vi "Editor.vi"(9 "Editor Events":T11, 11 "VIDoc Settings - Confluence In":refnum<class "VIDoc Settings - Confluence.lvclass">) -> (3 "VIDoc Settings - Confluence Out":refnum<class "VIDoc Settings - Confluence.lvclass">)   [LabVIEW 2023, in "VIDoc Printer - Confluence.lvlib" / "VIDoc Settings - Confluence.lvclass"]
uses:
  VIDoc Settings - Confluence.lvclass
  Interfaces/VIDoc Editor/Editor Events Cluster.ctl
  Confluence Connection Settings.ctl
  Class Info Column.ctl
  VI Info Column.ctl
  Control Info Column.ctl
  VIDoc Settings - Confluence.lvclass/VIDoc Settings - Confluence.ctl
  <userlib>/_PetranWay/LabVIEW Confluence API/Source/Data Center/Confluence Data Center/Confluence Data Center.lvclass
  C:/Program Files/National Instruments/LabVIEW 2023/user.lib/_PetranWay/LabVIEW Confluence API/Source/Confluence/Confluence Connection/Confluence.lvclass
  <userlib>/_PetranWay/LabVIEW Confluence API/Source/Cloud/Confluence Cloud/Confluence Cloud.lvclass
  <userlib>/_PetranWay/LabVIEW Confluence API/Source/Data Center/Confluence Data Center/API/Construct Confluence Data Center From Cache.vi
  <userlib>/_PetranWay/LabVIEW Confluence API/Source/Cloud/Confluence Cloud/API/Construct Confluence Cloud From Cache.vi
  <userlib>/_PetranWay/LabVIEW Confluence API/Source/Confluence/Confluence Connection/Confluence.lvclass
  Interfaces/VIDoc Editor/VIDocEditor.lvclass
panel:
  in  "Sections Tabs":T1(tab)
  out "Connection?":bool
  in  "Test Confluence Connection":bool
  in  "Sortable Tables":bool=TRUE
  in  "Confluence Connection Settings":T2
  in  "Expand Structures":T3={"VI Member"={"By Folder Expand"=TRUE, "By Tree Expand"=TRUE, "By List Expand"=TRUE, "Methods Expand"=TRUE, "Controls Expand"=TRUE}, "Control Member"={"By Folder Expand"=TRUE, "By Tree Expand"=TRUE, "By List Expand"=TRUE, "Controls Expand"=TRUE}, "Interface"={"List Expand"=TRUE, "Controls Expand"=TRUE, "Methods Expand"=TRUE, "Inheritance Expand"=TRUE}, "Library"={"By Folder Expand"=TRUE, "By Tree Expand"=TRUE, "By List Expand"=TRUE, "Controls Expand"=TRUE, "Methods Expand"=TRUE, "Inheritance Expand"=TRUE}, "Class"={"By Folder Expand"=TRUE, "By Tree Expand"=TRUE, "By List Expand"=TRUE, "CPD Expand"=TRUE, "Controls Expand"=TRUE, "Methods Expand"=TRUE, "Set Accessors Expand"=TRUE, "Get Accessors Expand"=TRUE, "Inheritance Expand"=TRUE}}
  in  "Table Column Ordering":T4(tab)
  in  "Class List":T6
  in  "Library List":T6
  in  "Method List":T8
  in  "Interface Methods":T8
  in  "Library Methods":T8
  in  "Class Methods":T8
  in  "LLB Methods":T8
  in  "UI Methods":T8
  in  "Library Control Files":T8
  in  "Control FP":T10
  # "Effects:\nClass - By List\nClass - Inheritance Parent Class\nClass - Inheritance Parent Interfaces\nInterface - By List\nInterface - Inheritance Parent Interfaces"
  # "Effects:\nClass - Inheritance Parent Libraries\nLibrary - By List"
  # "Effects:\nControls - By List\nUI - By List"
  # "Effects:\nInterface - Methods"
  # "Effects:\nLibrary - Methods"
  # "Effects:\nGet Accessors\nSet Accessors\nClass - Methods"
  # "Effects:\nLLB - Methods"
  # "Effects:\nUI - Method Details"
  # "Effects:\nClass - Controls\nInterface - Controls\nLibrary - Controls\nLLB - Controls"
  # "Effects:\nClass - CPD\nControls - Controls\nUI - Controls"
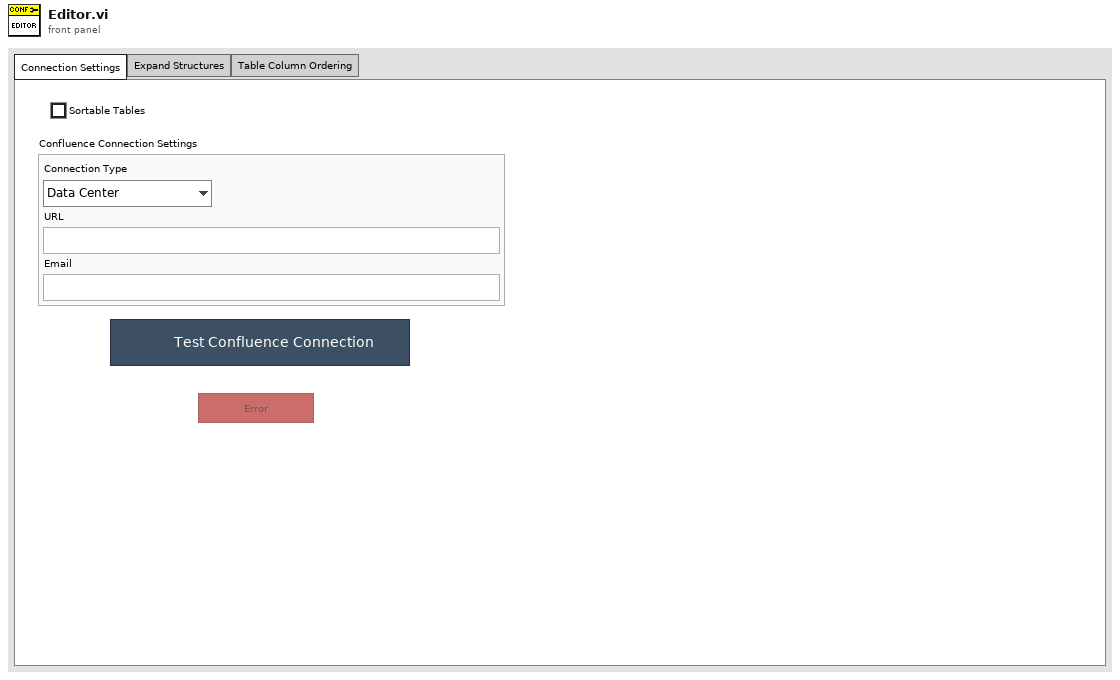
[diagram p1: front panel]
types:
  T1 = enum32{"Connection Settings", "Expand Structures", "Table Column Ordering"}
  T2 = typedef "VIDoc Printer - Confluence.lvlib/VIDoc Settings - Confluence.lvclass/Confluence Connection Settings.ctl" = cluster{"Connection Type":enum16{"Data Center", "Cloud"}, "URL":string, "Email":string}
  T3 = cluster{"VI Member":cluster{"By Folder Expand":bool, "By Tree Expand":bool, "By List Expand":bool, "Methods Expand":bool, "Controls Expand":bool}, "Control Member":cluster{"By Folder Expand":bool, "By Tree Expand":bool, "By List Expand":bool, "Controls Expand":bool}, "Interface":cluster{"List Expand":bool, "Controls Expand":bool, "Methods Expand":bool, "Inheritance Expand":bool}, "Library":cluster{"By Folder Expand":bool, "By Tree Expand":bool, "By List Expand":bool, "Controls Expand":bool, "Methods Expand":bool, "Inheritance Expand":bool}, "Class":cluster{"By Folder Expand":bool, "By Tree Expand":bool, "By List Expand":bool, "CPD Expand":bool, "Controls Expand":bool, "Methods Expand":bool, "Set Accessors Expand":bool, "Get Accessors Expand":bool, "Inheritance Expand":bool}}
  T4 = enum32{"Class List", "Library List", "Methods List", "Interface Methods", "Library Methods", "Class Methods", "LLB Methods", "UI Methods", "Library Control Files", "Font Panel Controls"}
  T5 = typedef "VIDoc Printer - Confluence.lvlib/VIDoc Settings - Confluence.lvclass/Class Info Column.ctl" = enum16{"Image", "Name", "Description", "Version", "Last Change", "Author", "Commit Hash", "Branch", "Qualified Name", "TransferMustOverrides", "ChildRefsRestricted"}
  T6 = cluster{"Minimal":T5[], "Standard":T5[], "Full":T5[]}
  T7 = typedef "VIDoc Printer - Confluence.lvlib/VIDoc Settings - Confluence.lvclass/VI Info Column.ctl" = enum16{"Name", "Conpane", "BD", "FP", "VI Icon", "Description", "Reentrant", "Inline", "Auto Error", "Compiled", "Code Complexity", "Data Size", "Debug", "Priority", "Rev", "Minimum Size", "Title", "FP Behavior", "FP Closeable", "Author", "Commit Hash", "Last Change", "Branch", "Scope", "Type", "Dispatch", "Must Override", "Must Use Parent", "Structure Tree"}
  T8 = cluster{"Minimal":T7[], "Standard":T7[], "Full":T7[]}
  T9 = typedef "VIDoc Printer - Confluence.lvlib/VIDoc Settings - Confluence.lvclass/Control Info Column.ctl" = enum16{"Image", "Name", "Description", "Caption", "Tip Strip", "Data Type", "Key Toggle"}
  T10 = cluster{"Minimal":T9[], "Standard":T9[], "Full":T9[]}
  T11 = typedef "VIDocEditor.lvclass/Editor Events Cluster.ctl" = cluster{"Close":refnum<user-event>, "Revert":refnum<user-event>, "Save":refnum<user-event>, "Changes?":refnum<user-event>}
  T12 = enum8{"Enabled", "Disabled", "Disabled and Grayed Out"}
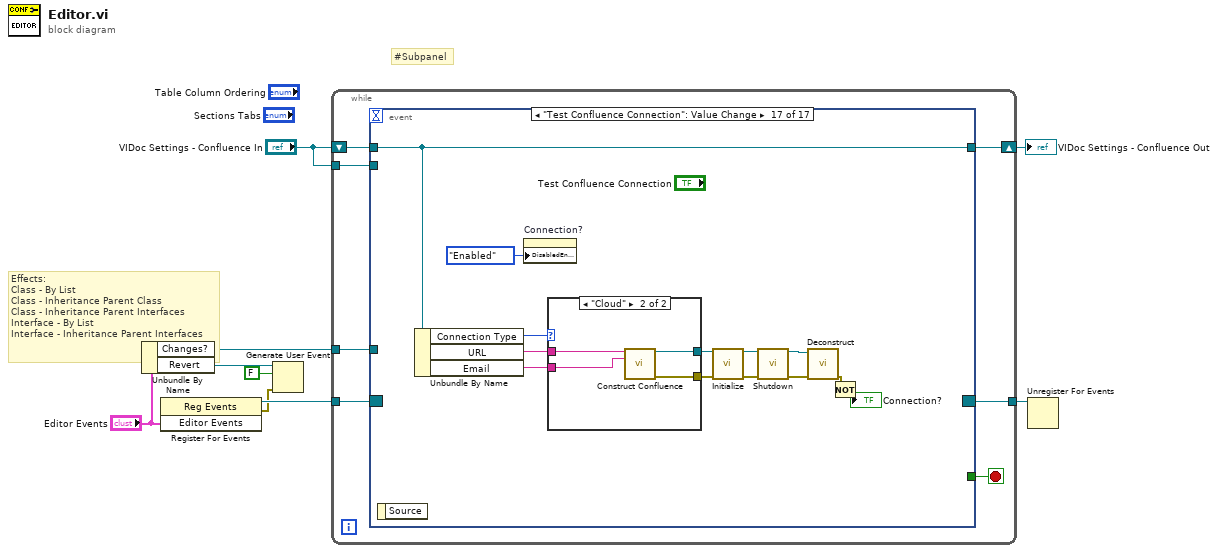
[diagram p0: block diagram]
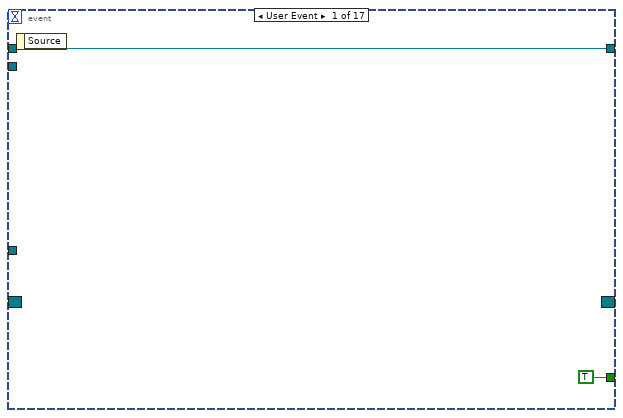
[diagram p2: hidden frame]
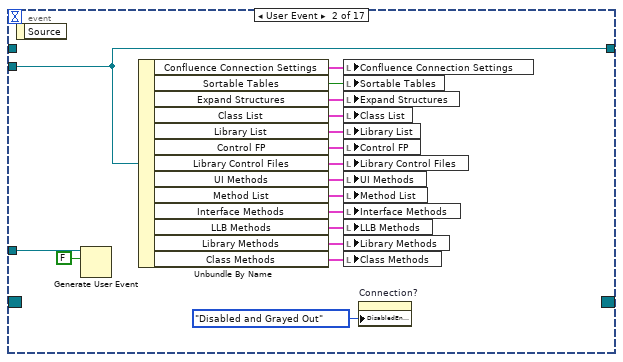
[diagram p3: hidden frame]
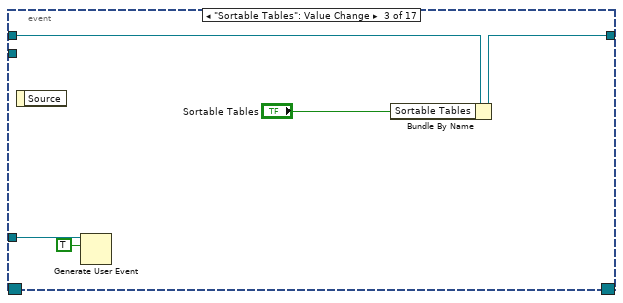
[diagram p4: hidden frame]
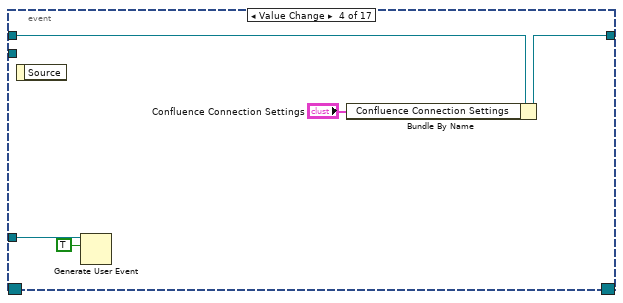
[diagram p5: hidden frame]
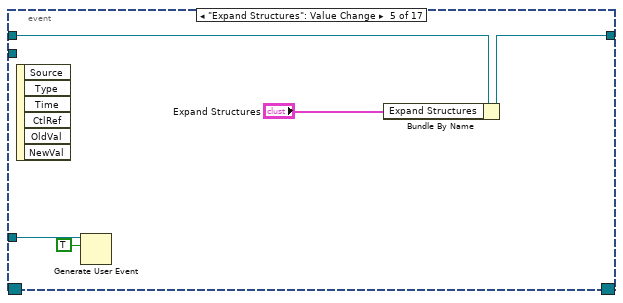
[diagram p6: hidden frame]
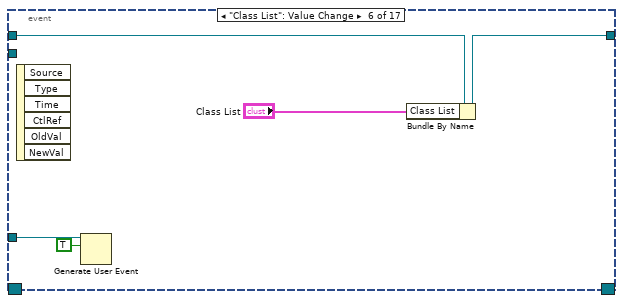
[diagram p7: hidden frame]
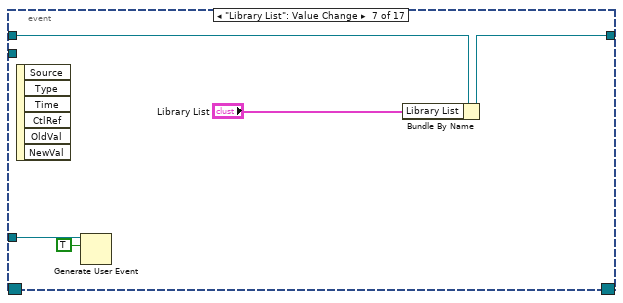
[diagram p8: hidden frame]
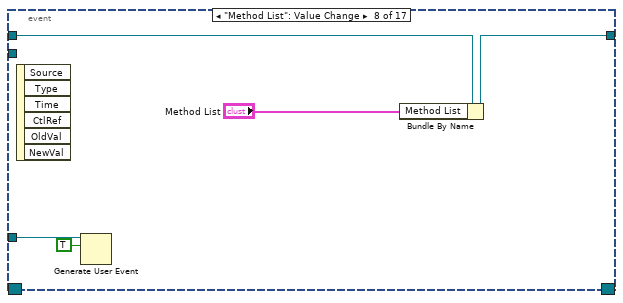
[diagram p9: hidden frame]
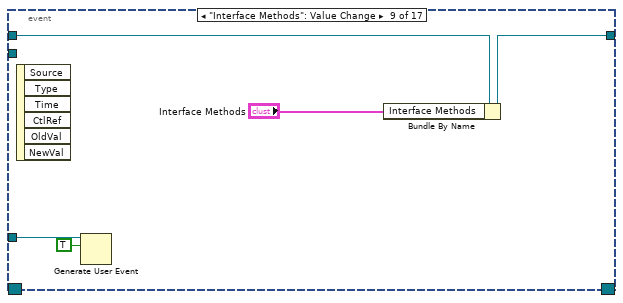
[diagram p10: hidden frame]
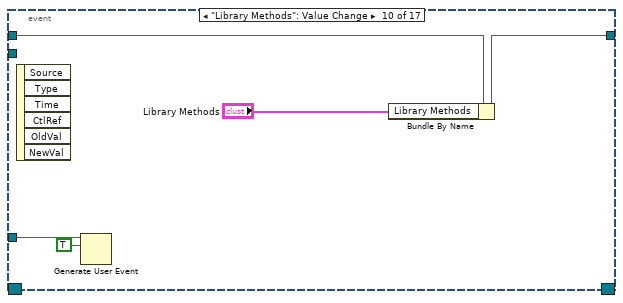
[diagram p11: hidden frame]
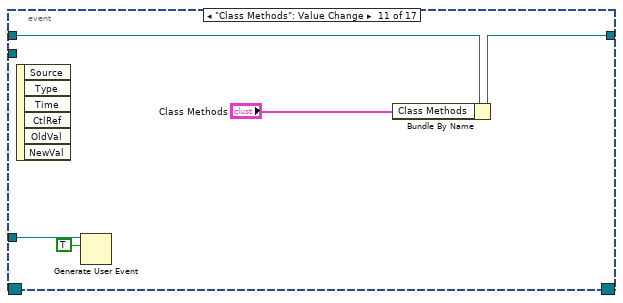
[diagram p12: hidden frame]
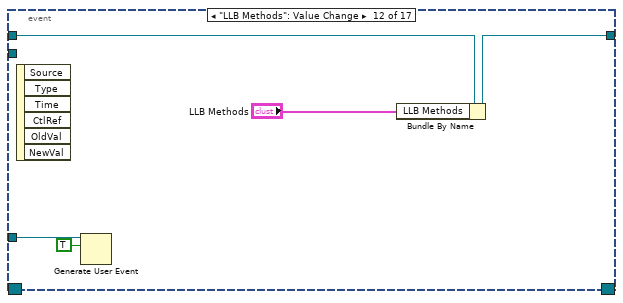
[diagram p13: hidden frame]
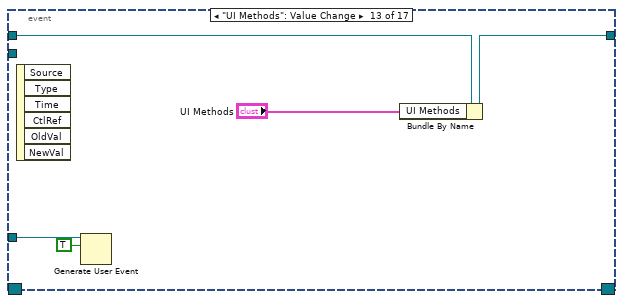
[diagram p14: hidden frame]
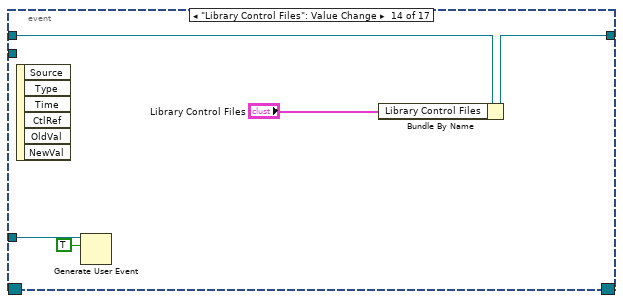
[diagram p15: hidden frame]
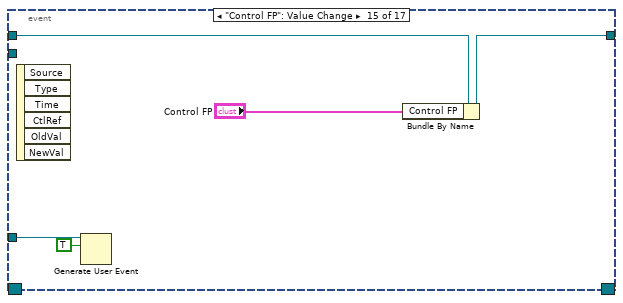
[diagram p16: hidden frame]
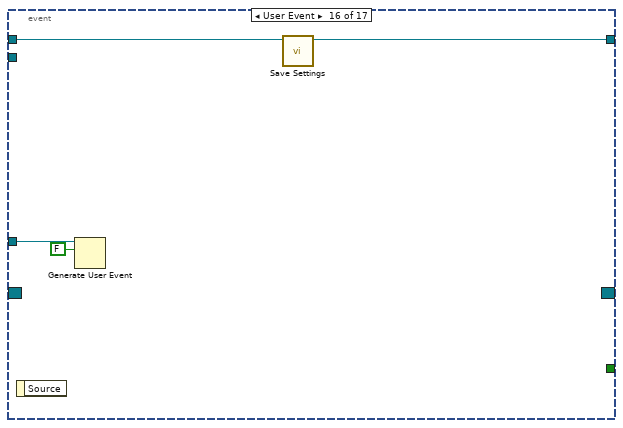
[diagram p17: hidden frame]
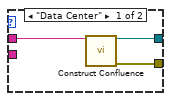
[diagram p18: hidden frame]
diagram:
  # "#Subpanel"
  # "Effects:\nClass - By List\nClass - Inheritance Parent Class\nClass - Inheritance Parent Interfaces\nInterface - By List\nInterface - Inheritance Parent Interfaces"
  n1 = Unbundle By Name("Editor Events") -> ("Changes?"=w1:refnum<user-event>, "Revert"=w4:refnum<user-event>)
  n2 = register-events("Editor Events") -> (reference out=w9:refnum<event-registration>, error out=w2:errorcluster)  [unwired: 2 in]
  n3 = Generate User Event(user event=w4, event data cluster=FALSE ("event data"), error in=w2) -> ()  [unwired: 1 in, 2 out]
  n4 = while {
    shift-right: [w14] -> w7
    shift-left: "VIDoc Settings - Confluence In" -> [w16]
    tunnel: w9 -> [w15]
    tunnel: [w12] -> w8
    tunnel: "VIDoc Settings - Confluence In" -> [w11]
    tunnel: w1 -> [w10]
    stop <- w13 stop-if-true
    n5 = event shown="[16] \"Test Confluence Connection\": Value Change" {
      selector: w15 -> [_ _ _ _ _ _ _ _ _ _ _ _ _ _ _ _ _]
      dyn-events: [_ _ _ _ _ _ _ _ _ _ _ _ _ _ _ _ _] -> w12
      timeout: _ -> [_ _ _ _ _ _ _ _ _ _ _ _ _ _ _ _ _]
      tunnel: w16 -> [w18 _ w40 w45 w50 w55 w60 w65 w70 w75 w80 w85 w90 w95 w100 w103 w114]
      tunnel: [w18 w35 w39 w44 w49 w54 w59 w64 w69 w74 w79 w84 w89 w94 w99 w104 w114] -> w14
      tunnel: [TRUE _ _ _ _ _ _ _ _ _ _ _ _ _ _ _ _] -> w13
      tunnel: w11 -> [_ w35 _ _ _ _ _ _ _ _ _ _ _ _ _ _ _]
      tunnel: w10 -> [_ w33 w37 w42 w47 w52 w57 w62 w67 w72 w77 w82 w87 w92 w97 w101 _]
      event User Event {
        n6 = event-data() -> ()  [unwired: 1 in, 1 out]
      }
      event User Event {
        n7 = event-data() -> ()  [unwired: 1 in, 1 out]
        n8 = Generate User Event(user event=w33, event data cluster=FALSE ("event data")) -> ()  [unwired: 2 in, 2 out]
        n9 = Unbundle By Name(w35) -> ("Confluence Connection Settings"=w32:T2, "Sortable Tables"=w31:bool, "Expand Structures"=w30:T3, "Class List"=w29:T6, "Library List"=w28:T6, "Control FP"=w27:T10, "Library Control Files"=w26:T8, "UI Methods"=w25:T8, "Method List"=w24:T8, "Interface Methods"=w23:T8, "LLB Methods"=w22:T8, "Library Methods"=w21:T8, "Class Methods"=w20:T8)
        n10 = local write "Confluence Connection Settings"(w32) -> ()
        n11 = local write "Sortable Tables"(w31) -> ()
        n12 = local write "Expand Structures"(w30) -> ()
        n13 = local write "Class List"(w29) -> ()
        n14 = local write "Library List"(w28) -> ()
        n15 = local write "Control FP"(w27) -> ()
        n16 = local write "Library Control Files"(w26) -> ()
        n17 = local write "UI Methods"(w25) -> ()
        n18 = local write "Method List"(w24) -> ()
        n19 = local write "Interface Methods"(w23) -> ()
        n20 = local write "LLB Methods"(w22) -> ()
        n21 = local write "Library Methods"(w21) -> ()
        n22 = local write "Class Methods"(w20) -> ()
        n23 = property on="Connection?" class="Bool"("DisabledEnum"=T12."Disabled and Grayed Out" ("Disabled")) -> ()  [unwired: 2 in, 2 out]
      }
      event "Sortable Tables": Value Change {
        n24 = event-data() -> ()  [unwired: 1 in, 1 out]
        n25 = Generate User Event(user event=w37, event data cluster=TRUE ("event data")) -> ()  [unwired: 2 in, 2 out]
        n26 = Bundle By Name(cluster=w40, "Sortable Tables"="Sortable Tables") -> (w39:refnum<class "VIDoc Settings - Confluence.lvclass">)
      }
      event Value Change {
        n27 = event-data() -> ()  [unwired: 1 in, 1 out]
        n28 = Generate User Event(user event=w42, event data cluster=TRUE ("event data")) -> ()  [unwired: 2 in, 2 out]
        n29 = Bundle By Name(cluster=w45, "Confluence Connection Settings"="Confluence Connection Settings") -> (w44:refnum<class "VIDoc Settings - Confluence.lvclass">)
      }
      event "Expand Structures": Value Change {
        n30 = event-data() -> ()  [unwired: 1 in, 6 out]
        n31 = Generate User Event(user event=w47, event data cluster=TRUE ("event data")) -> ()  [unwired: 2 in, 2 out]
        n32 = Bundle By Name(cluster=w50, "Expand Structures"="Expand Structures") -> (w49:refnum<class "VIDoc Settings - Confluence.lvclass">)
      }
      event "Class List": Value Change {
        n33 = event-data() -> ()  [unwired: 1 in, 6 out]
        n34 = Generate User Event(user event=w52, event data cluster=TRUE ("event data")) -> ()  [unwired: 2 in, 2 out]
        n35 = Bundle By Name(cluster=w55, "Class List"="Class List") -> (w54:refnum<class "VIDoc Settings - Confluence.lvclass">)
      }
      event "Library List": Value Change {
        n36 = event-data() -> ()  [unwired: 1 in, 6 out]
        n37 = Generate User Event(user event=w57, event data cluster=TRUE ("event data")) -> ()  [unwired: 2 in, 2 out]
        n38 = Bundle By Name(cluster=w60, "Library List"="Library List") -> (w59:refnum<class "VIDoc Settings - Confluence.lvclass">)
      }
      event "Method List": Value Change {
        n39 = event-data() -> ()  [unwired: 1 in, 6 out]
        n40 = Generate User Event(user event=w62, event data cluster=TRUE ("event data")) -> ()  [unwired: 2 in, 2 out]
        n41 = Bundle By Name(cluster=w65, "Method List"="Method List") -> (w64:refnum<class "VIDoc Settings - Confluence.lvclass">)
      }
      event "Interface Methods": Value Change {
        n42 = event-data() -> ()  [unwired: 1 in, 6 out]
        n43 = Generate User Event(user event=w67, event data cluster=TRUE ("event data")) -> ()  [unwired: 2 in, 2 out]
        n44 = Bundle By Name(cluster=w70, "Interface Methods"="Interface Methods") -> (w69:refnum<class "VIDoc Settings - Confluence.lvclass">)
      }
      event "Library Methods": Value Change {
        n45 = event-data() -> ()  [unwired: 1 in, 6 out]
        n46 = Generate User Event(user event=w72, event data cluster=TRUE ("event data")) -> ()  [unwired: 2 in, 2 out]
        n47 = Bundle By Name(cluster=w75, "Library Methods"="Library Methods") -> (w74:refnum<class "VIDoc Settings - Confluence.lvclass">)
      }
      event "Class Methods": Value Change {
        n48 = event-data() -> ()  [unwired: 1 in, 6 out]
        n49 = Generate User Event(user event=w77, event data cluster=TRUE ("event data")) -> ()  [unwired: 2 in, 2 out]
        n50 = Bundle By Name(cluster=w80, "Class Methods"="Class Methods") -> (w79:refnum<class "VIDoc Settings - Confluence.lvclass">)
      }
      event "LLB Methods": Value Change {
        n51 = event-data() -> ()  [unwired: 1 in, 6 out]
        n52 = Generate User Event(user event=w82, event data cluster=TRUE ("event data")) -> ()  [unwired: 2 in, 2 out]
        n53 = Bundle By Name(cluster=w85, "LLB Methods"="LLB Methods") -> (w84:refnum<class "VIDoc Settings - Confluence.lvclass">)
      }
      event "UI Methods": Value Change {
        n54 = event-data() -> ()  [unwired: 1 in, 6 out]
        n55 = Generate User Event(user event=w87, event data cluster=TRUE ("event data")) -> ()  [unwired: 2 in, 2 out]
        n56 = Bundle By Name(cluster=w90, "UI Methods"="UI Methods") -> (w89:refnum<class "VIDoc Settings - Confluence.lvclass">)
      }
      event "Library Control Files": Value Change {
        n57 = event-data() -> ()  [unwired: 1 in, 6 out]
        n58 = Generate User Event(user event=w92, event data cluster=TRUE ("event data")) -> ()  [unwired: 2 in, 2 out]
        n59 = Bundle By Name(cluster=w95, "Library Control Files"="Library Control Files") -> (w94:refnum<class "VIDoc Settings - Confluence.lvclass">)
      }
      event "Control FP": Value Change {
        n60 = event-data() -> ()  [unwired: 1 in, 6 out]
        n61 = Generate User Event(user event=w97, event data cluster=TRUE ("event data")) -> ()  [unwired: 2 in, 2 out]
        n62 = Bundle By Name(cluster=w100, "Control FP"="Control FP") -> (w99:refnum<class "VIDoc Settings - Confluence.lvclass">)
      }
      event User Event {
        n63 = event-data() -> ()  [unwired: 1 in, 1 out]
        n64 = Generate User Event(user event=w101, event data cluster=FALSE ("event data")) -> ()  [unwired: 2 in, 2 out]
        n65 = call-dynamic "Save Settings.vi"("VIDoc Settings - Confluence In"=w103) -> ("VIDoc Settings - Confluence Out"=w104:refnum<class "VIDoc Settings - Confluence.lvclass">)  [unwired: 9 in, 1 out]
      }
      event "Test Confluence Connection": Value Change {
        n66 = event-data() -> ()  [unwired: 1 in, 1 out]
        n67 = Unbundle By Name(w114) -> ("Connection Type"=w117:enum16{"Data Center", "Cloud"}, "URL"=w116:string, "Email"=w115:string)
        n68 = property on="Connection?" class="Bool"("DisabledEnum"=T12."Enabled" ("Disabled")) -> ()  [unwired: 2 in, 2 out]
        n69 = case shown="\"Cloud\"" w117 {
          tunnel: [w120 w124] -> w113
          tunnel: [w119 w123] -> w112
          tunnel: w116 -> [w118 w122]
          tunnel: w115 -> [_ w121]
          frame "Data Center" {
            n70 = call-poly <userlib>:"Construct Confluence.vi"("Server URL"=w118) -> ("Confluence Data Center out"=w119:refnum<class "Confluence Data Center.lvclass">, "error out"=w120:errorcluster)  [unwired: 11 in, 2 out]
          }
          frame "Cloud" {
            n71 = call-poly <userlib>:"Construct Confluence.vi"("Organization Name (https://[Organization Name].atlassian.net]"=w122, "Email Address"=w121) -> ("Confluence Cloud out"=w123:refnum<class "Confluence Cloud.lvclass">, "error out"=w124:errorcluster)  [unwired: 10 in, 2 out]
          }
        }
        n72 = call-dynamic "Initialize.vi"("Confluence in"=w112, "error in (no error)"=w113) -> ("Confluence out"=w111:refnum<class "Confluence.lvclass">, "error out"=w110:errorcluster)  [unwired: 12 in]
        n73 = call-dynamic "Shutdown.vi"("Confluence in"=w111, "error in (no error)"=w110) -> ("Confluence out"=w109:refnum<class "Confluence.lvclass">, "error out"=w108:errorcluster)  [unwired: 12 in]
        n74 = call-dynamic "Deconstruct.vi"("error in (no error)"=w108, "Confluence in"=w109) -> ("error out"=w106:errorcluster)  [unwired: 9 in]
        n75 = Not(x=w106) -> (.not. x?=→"Connection?":bool)
      }
    }
  }
  "VIDoc Settings - Confluence Out" <- w7
  n76 = Unregister For Events(event registration refnum=w8) -> ()  [unwired: 1 in, 1 out]
